vi "SPARK Get Limit Switch Status.vi"   [LabVIEW 2023]
doc: "Get the status of a limit switch connected to the data port of the SPARK."
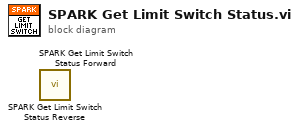
[diagram p0: block diagram]
diagram:
  n1 = call "SPARK Get Limit Switch Status Reverse.vi"() -> ()  [unwired: 8 in, 4 out]
  n2 = call "SPARK Get Limit Switch Status Forward.vi"() -> ()  [unwired: 8 in, 4 out]
